vi "Flat Sequence.vi"() -> ()   [LabVIEW 2016]
panel:
  out "Boolean 3":bool
  out "Boolean 2":bool
  out "Boolean":bool
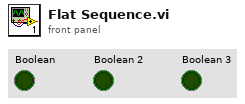
[diagram p1: front panel]
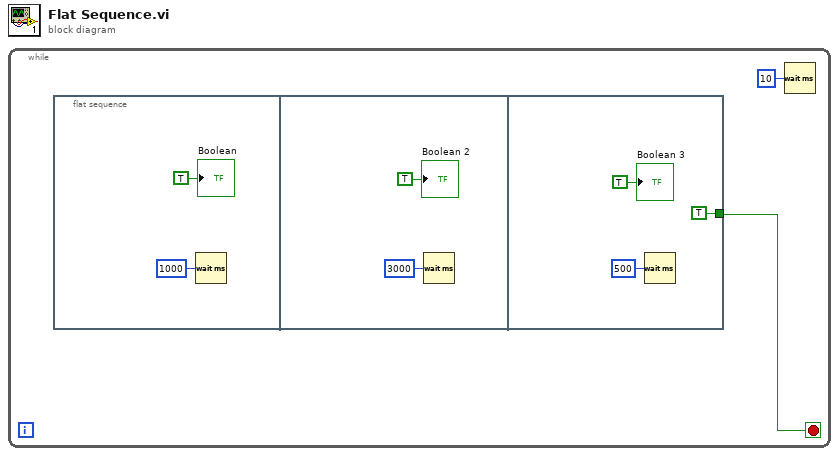
[diagram p0: block diagram]
diagram:
  n1 = while {
    stop <- w1 stop-if-true
    n2 = flat-sequence {
      tunnel: [TRUE] -> w1
      frame #0 {
        n3 = Wait (ms)(milliseconds to wait=u32 1000) -> ()  [unwired: 1 out]
        "Boolean" <- TRUE ("Boolean")
      }
      frame #1 {
        n4 = Wait (ms)(milliseconds to wait=u32 3000) -> ()  [unwired: 1 out]
        "Boolean 2" <- TRUE ("Boolean 2")
      }
      frame #2 {
        n5 = Wait (ms)(milliseconds to wait=u32 500) -> ()  [unwired: 1 out]
        "Boolean 3" <- TRUE ("Boolean 3")
      }
    }
    n6 = Wait (ms)(milliseconds to wait=u32 10) -> ()  [unwired: 1 out]
  }
